vi "Array 2 Cartesian Point.vi"(3 "Array":dbl[](array[numeric])) -> (0 "Cart Disp":T1)   [LabVIEW 2013]
uses:
  Metadata/Cartesian Point.ctl
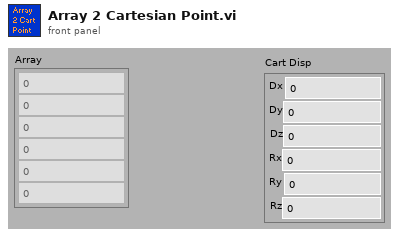
[diagram p1: front panel]
types:
  T1 = typedef "Cartesian Point.ctl" = cluster{"Dx":dbl, "Dy":dbl, "Dz":dbl, "Rx":dbl, "Ry":dbl, "Rz":dbl}
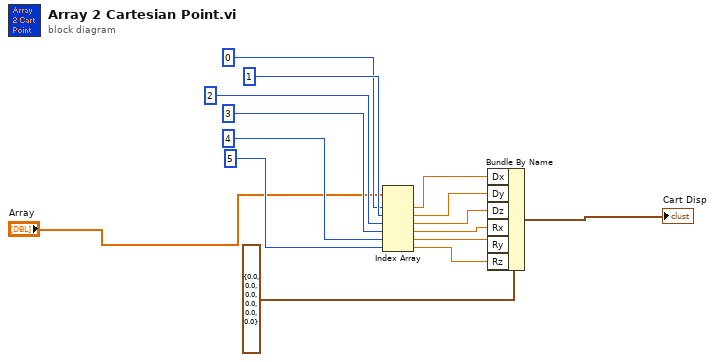
[diagram p0: block diagram]
diagram:
  n1 = Index Array(array="Array", index #1=0 ("index"), index #2=1 ("index"), index #3=2 ("index"), index #4=3 ("index"), index #5=4 ("index"), index #6=5 ("index")) -> (element #1=w3:dbl, element #2=w4:dbl, element #3=w5:dbl, element #4=w6:dbl, element #5=w7:dbl, element #6=w8:dbl)
  n2 = Bundle By Name(cluster=T1 {"Dx"=0.0, "Dy"=0.0, "Dz"=0.0, "Rx"=0.0, "Ry"=0.0, "Rz"=0.0} ("Maximum \nDisplacement\nIncrement"), "Dx"=w3, "Dy"=w4, "Dz"=w5, "Rx"=w6, "Ry"=w7, "Rz"=w8) -> (→"Cart Disp":T1)
